vi "Get Base Protocol.vi"(8 "error in (no error)":errorcluster, 11 "RS232 to GPIB ConvBox in":refnum<class "RSxxx to GPIB ConvBox.lvclass">) -> (0 "error out":errorcluster, 2 "Protocol out":T1, 3 "RS232 to GPIB ConvBox out":refnum<class "RSxxx to GPIB ConvBox.lvclass">)   [LabVIEW 2019, in "Protocols.lvlib" / "RSxxx to GPIB ConvBox.lvclass"]
uses:
  RSxxx to GPIB ConvBox.lvclass
  Protocol Parent/Types/Base Protocol Type.ctl
  Protocol Parent/Protocol Parent.lvclass
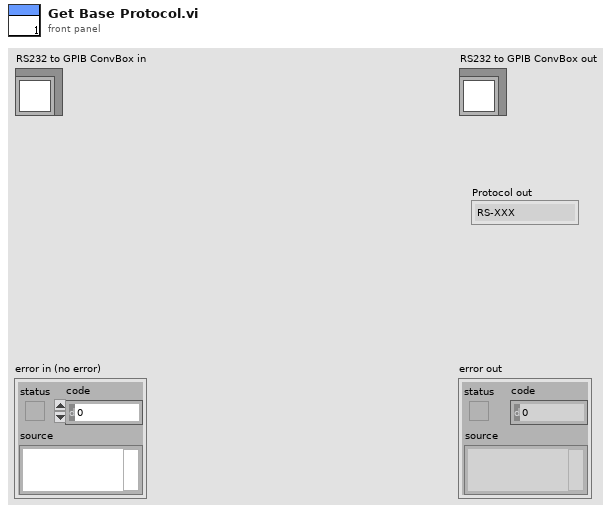
[diagram p1: front panel]
types:
  T1 = typedef "Protocols.lvlib/Protocol Parent.lvclass/Base Protocol Type.ctl" = enum16{"RS-XXX", "VISA", "TCPIP", "UDP", "GPIB ConvBox"}
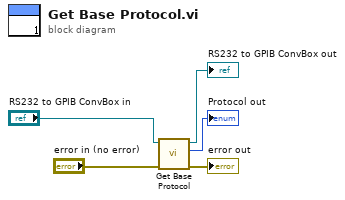
[diagram p0: block diagram]
diagram:
  n1 = call-parent "Get Base Protocol.vi"("error in (no error)"="error in (no error)", "Protocol Parent in"="RS232 to GPIB ConvBox in") -> ("error out"=→"error out":errorcluster, "Protocol out"=→"Protocol out":T1, "Protocol Parent out"=→"RS232 to GPIB ConvBox out":refnum<class "RSxxx to GPIB ConvBox.lvclass">)  [unwired: 7 in]
